vi "Configure Window Trigger.vi"(0 "VISA resource name":refnum<visa-resource-name>, 1 "Low Boundary":dbl, 5 "Function":u16(ring) items=["Voltage: DC", "Voltage: AC", "Current: DC", "Current: AC", "2W Resistance", "4W Resistance", "Diode", "Capacitance", "Temperature", "Continuity", "Frequency", "Period", "Ratio", "Digitize Voltage", "Digitize Current"], 7 "Direction":u16(ring) items=["Enter", "Leave"], 9 "High Boundary":dbl=1.0, 11 "error in (no error)":errorcluster, 12 "HF Rejection":bool=TRUE) -> (4 "VISA resource name out":refnum<visa-resource-name>, 15 "error out":errorcluster)   [LabVIEW 2021, in "Keithley DMM7510.lvlib"]
doc: "This VI sets the slope and level of the analog edge trigger. This also enables or disables the high frequency rejection for analog trigger."
uses:
  Keithley DMM7510.lvlib
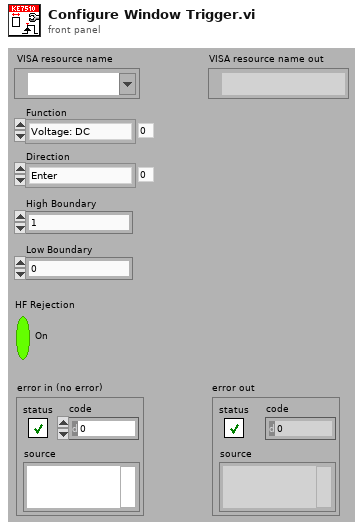
[diagram p1: front panel]
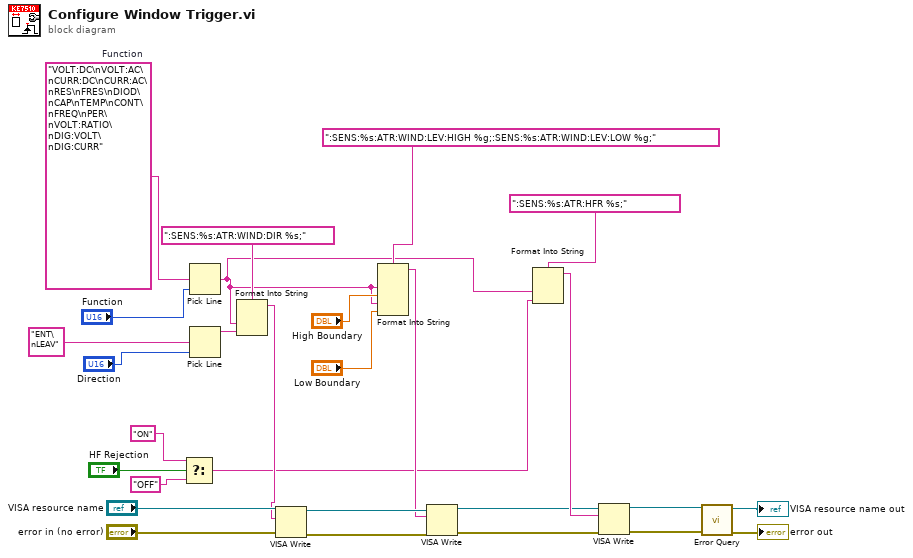
[diagram p0: block diagram]
diagram:
  w24 = "VOLT:DC\nVOLT:AC\nCURR:DC\nCURR:AC\nRES\nFRES\nDIOD\nCAP\nTEMP\nCONT\nFREQ\nPER\nVOLT:RATIO\nDIG:VOLT\nDIG:CURR"  # Function
  n1 = Select(t="ON" ("format string"), s="HF Rejection", f="OFF" ("format string")) -> (s? t:f=w4:string)
  n2 = Pick Line(multi-line string=w24, line index="Function") -> (output string=w3:string)  [unwired: 1 in]
  n3 = Pick Line(multi-line string="ENT\nLEAV", line index="Direction") -> (output string=w22:string)  [unwired: 1 in]
  n4 = Format Into String(format string=":SENS:%s:ATR:WIND:DIR %s;", w3, w22) -> (resulting string=w16:string)  [unwired: 2 in, 1 out]
  n5 = VISA Write(VISA resource name="VISA resource name", write buffer=w16, error in (no error)="error in (no error)") -> (VISA resource name out=w15:refnum<visa-resource-name>, error out=w14:errorcluster)  [unwired: 1 out]
  n6 = Format Into String(format string=":SENS:%s:ATR:WIND:LEV:HIGH %g;:SENS:%s:ATR:WIND:LEV:LOW %g;", w3, "High Boundary", w3, "Low Boundary") -> (resulting string=w13:string)  [unwired: 2 in, 1 out]
  n7 = VISA Write(VISA resource name=w15, write buffer=w13, error in (no error)=w14) -> (VISA resource name out=w8:refnum<visa-resource-name>, error out=w5:errorcluster)  [unwired: 1 out]
  n8 = Format Into String(format string=":SENS:%s:ATR:HFR %s;", w3, w4) -> (resulting string=w9:string)  [unwired: 2 in, 1 out]
  n9 = VISA Write(VISA resource name=w8, write buffer=w9, error in (no error)=w5) -> (VISA resource name out=w7:refnum<visa-resource-name>, error out=w6:errorcluster)  [unwired: 1 out]
  n10 = call "Error Query.vi"("error in (no error)"=w6, "VISA resource name"=w7) -> ("error out"=→"error out":errorcluster, "VISA resource name out"=→"VISA resource name out":refnum<visa-resource-name>)  [unwired: 6 in, 2 out]
